vi "Unregister All Controls.vi"(8 "error in (no error)":errorcluster, 11 "SlideEngine.lvclass In":refnum<class "SlideEngine.lvclass">) -> (0 "error out":errorcluster)   [LabVIEW 2012, in "SlideEngine.lvclass"]
doc: "This VI releases all the queue resources associated with registered controls which in turn causes the Consumer Daemons to exit."
uses:
  SlideEngine.lvclass
  SlideEngine.lvclass/SlideEngine.ctl
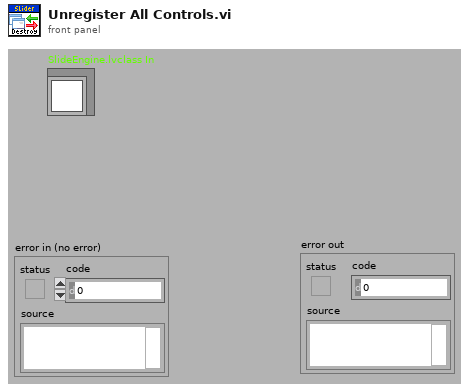
[diagram p1: front panel]
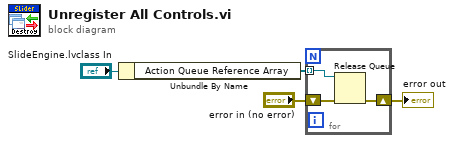
[diagram p0: block diagram]
diagram:
  n1 = Unbundle By Name("SlideEngine.lvclass In") -> ("Action Queue Reference Array"=w3:refnum<queue>[])
  n2 = for {
    tunnel: w3 -> [w7] mode=indexing
    shift-right: [w5] -> w1
    shift-left: "error in (no error)" -> [w6]
    n3 = Release Queue(queue=w7, error in (no error)=w6) -> (error out=w5:errorcluster)  [unwired: 3 out]
  }
  "error out" <- w1
